vi "Initialize.vi"(8 "error in (no error)":errorcluster, 10 "channels quantity":u8=1, 11 "AutoExp in":refnum<class "AutoExp.lvclass">) -> (0 "error out":errorcluster, 3 "AutoExp out":refnum<class "AutoExp.lvclass">)   [LabVIEW 2018, in "AutoExp.lvclass"]
uses:
  AutoExp.lvclass
  Channel/Channel.lvclass
  Channel/Channel.lvclass/Channel.ctl
  AutoExp.lvclass/AutoExp.ctl
panel:
  in  "Channel.lvclass":refnum<class "Channel.lvclass">
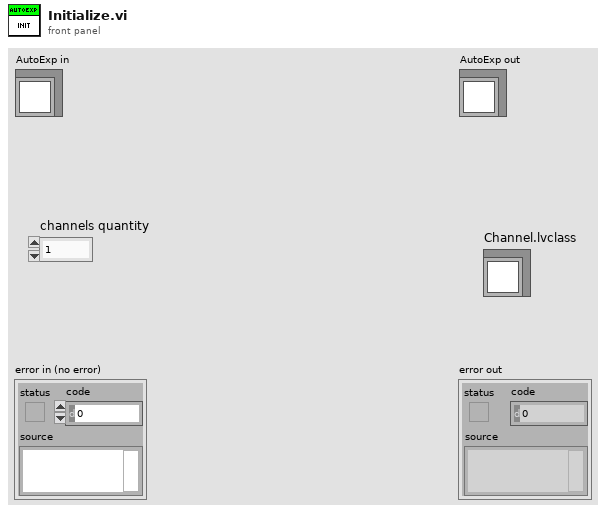
[diagram p1: front panel]
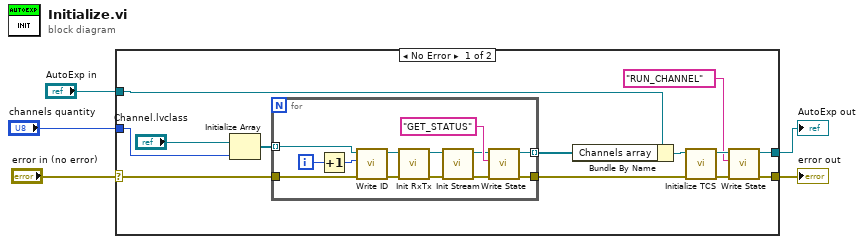
[diagram p0: block diagram]
diagram:
  n1 = case shown="No Error" "error in (no error)" {
    selector: "error in (no error)" -> [w16 w32]
    tunnel: [w9 w33] -> w3
    tunnel: "AutoExp in" -> [w15 w33]
    tunnel: [w8 w32] -> w2
    tunnel: "channels quantity" -> [w13 _]
    frame No Error {
      n2 = Initialize Array("Channel.lvclass", w13) -> (w17:refnum<class "Channel.lvclass">[])
      n3 = for {
        tunnel: w17 -> [w30] mode=indexing
        tunnel: w16 -> [w31]
        tunnel: [w20] -> w14 mode=indexing
        tunnel: [w19] -> w11
        i -> [w28]
        n4 = Increment(x=w28) -> (x+1=w29:i32)
        n5 = call "Write ID.vi"("error in (no error)"=w31, "ID"=w29, "Channel in"=w30) -> ("error out"=w26:errorcluster, "Channel out"=w27:refnum<class "Channel.lvclass">)  [unwired: 7 in]
        n6 = call "Init RxTx.vi"("error in (no error)"=w26, "Channel in"=w27) -> ("error out"=w24:errorcluster, "Channel out"=w25:refnum<class "Channel.lvclass">)  [unwired: 8 in]
        n7 = call "Init Stream.vi"("error in (no error)"=w24, "Channel in"=w25) -> ("error out"=w21:errorcluster, "Channel out"=w22:refnum<class "Channel.lvclass">)  [unwired: 8 in]
        n8 = call "Write State.vi"("error in (no error)"=w21, "State"="GET_STATUS" ("message"), "Channel in"=w22) -> ("error out"=w19:errorcluster, "Channel out"=w20:refnum<class "Channel.lvclass">)  [unwired: 7 in]
      }
      n9 = Bundle By Name(cluster=w15, "Channels array"=w14) -> (w12:refnum<class "AutoExp.lvclass">)
      n10 = call "Initialize TCS.vi"("error in (no error)"=w11, "AutoExp in"=w12) -> ("error out"=w7:errorcluster, "AutoExp out"=w10:refnum<class "AutoExp.lvclass">)  [unwired: 8 in]
      n11 = call "Write State.vi"("error in (no error)"=w7, "State"="RUN_CHANNEL", "AutoExp in"=w10) -> ("error out"=w8:errorcluster, "AutoExp out"=w9:refnum<class "AutoExp.lvclass">)  [unwired: 7 in]
    }
    frame Error {
    }
  }
  "error out" <- w2
  "AutoExp out" <- w3
